vi "2D DBL_Array_Sort.vi"(2 "Array in":dbl[][](array[numeric])) -> (6 "Array out":dbl[][](array[numeric]))   [LabVIEW 2020]
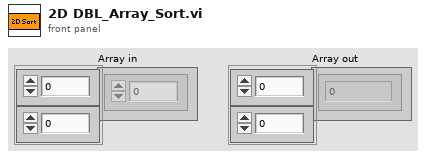
[diagram p1: front panel]
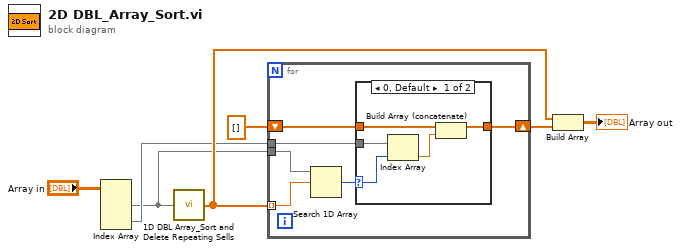
[diagram p0: block diagram]
diagram:
  n1 = Index Array(array="Array in") -> (element #1=w2:dbl[], element #2=w3:dbl[])  [unwired: 4 in]
  n2 = call "1D DBL Array_Sort and Delete Repeating Sells.vi"("1D DBL Array.In"=w2) -> ("1D DBL Array.Out"=w5:dbl[])  [unwired: 6 in]
  n3 = for {
    tunnel: w5 -> [w12] mode=indexing
    tunnel: w2 -> [w13]
    tunnel: w3 -> [w8]
    shift-right: [w9] -> w6
    shift-left: dbl[] [] ("subarray") -> [w10]
    n4 = Search 1D Array(1D array=w13, element=w12) -> (index of element=w11:i32)  [unwired: 1 in]
    n5 = case shown="0, Default" w11 {
      selector: w11 -> [w17 _]
      tunnel: w10 -> [w16 w19]
      tunnel: [w14 w19] -> w9
      tunnel: w8 -> [w18 _]
      frame 0, Default {
        n6 = Index Array(array=w18, index=w17) -> (element=w15:dbl)
        n7 = Build Array (concatenate)(w16, w15) -> (w14:dbl[])
      }
      frame -1 {
      }
    }
  }
  n8 = Build Array(w5, w6) -> (→"Array out":dbl[][])
